vi "luaL_typename.vi"(8 "error in (no error)":errorcluster, 10 "index":i32, 11 "lua_state_p":u64) -> (0 "error out":errorcluster, 2 "string":string, 3 "lua_state_p out":u64)   [LabVIEW 2020, in "lua.dll.lvlib"]
uses:
  lua.dll.lvlib
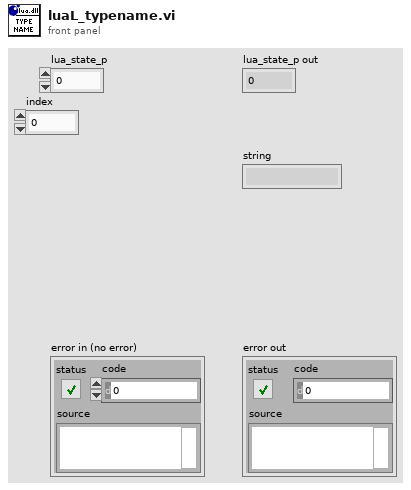
[diagram p1: front panel]
types:
  T1 = typedef "lua.dll.lvlib/lua_types.ctl" = i32
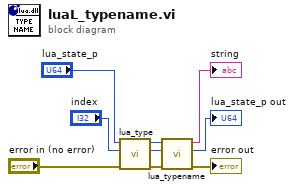
[diagram p0: block diagram]
diagram:
  n1 = call "lua_type.vi"("error in (no error)"="error in (no error)", "index"="index", "lua_state_p"="lua_state_p") -> ("error out"=w3:errorcluster, "lua type"=w1:T1, "lua_state_p out"=w2:u64)  [unwired: 6 in]
  n2 = call "lua_typename.vi"("error in (no error)"=w3, "lua type"=w1, "lua_state_p in"=w2) -> ("error out"=→"error out":errorcluster, "lua_state_p"=→"lua_state_p out":u64, "result"=→"string":string)  [unwired: 6 in]
